vi "OSF Upload File.vi"(6 "Append to Lab Notebook":bool, 7 "timeout":dbl=60.0 format="%#_6ps", 8 "error in":errorcluster, 9 "Token":string, 10 "Node":string="96bhe/files/", 11 "File name":path=path "C:/Data/April_2019/042419/sp0006_042419.tdms") -> (0 "error out":errorcluster)   [LabVIEW 2020]
uses:
  <vilib>/httpClient/PUTFile.vi
  <vilib>/httpClient/PUTBuffer.vi
  <vilib>/httpClient/LabVIEWHTTPClient.lvlib
panel:
  in  "Export Type":enum16{"Text", "Markdown"}(ring)
  out "Elapsed time":dbl format="%#_6ps"
  out "body 2":string
  out "body":string
  in  "OSF API URL":string="https://api.osf.io/v2/"
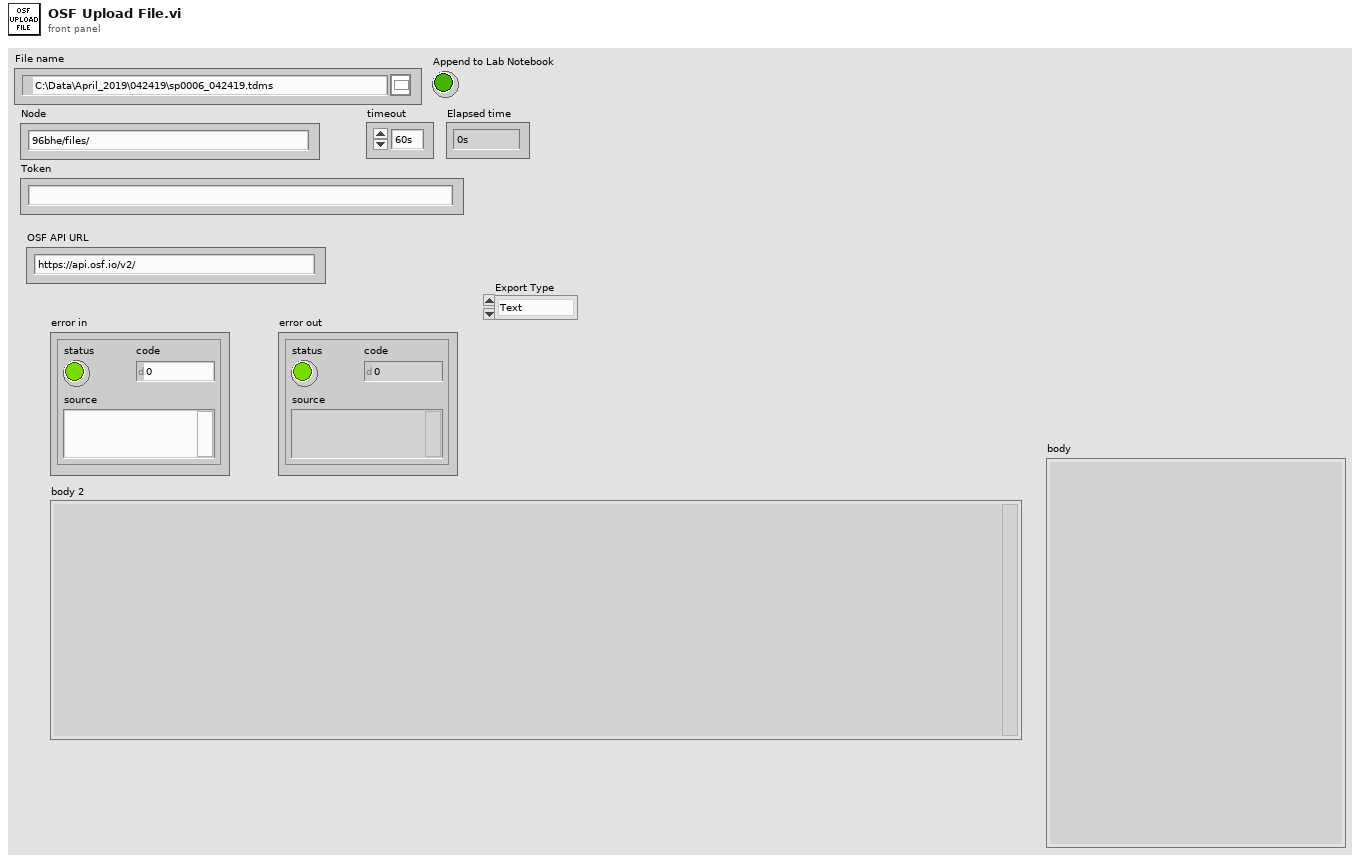
[diagram p1: front panel]
types:
  T1 = typedef "LabVIEWHTTPClient.lvlib/ClientHandle.ctl" = refnum<k1>
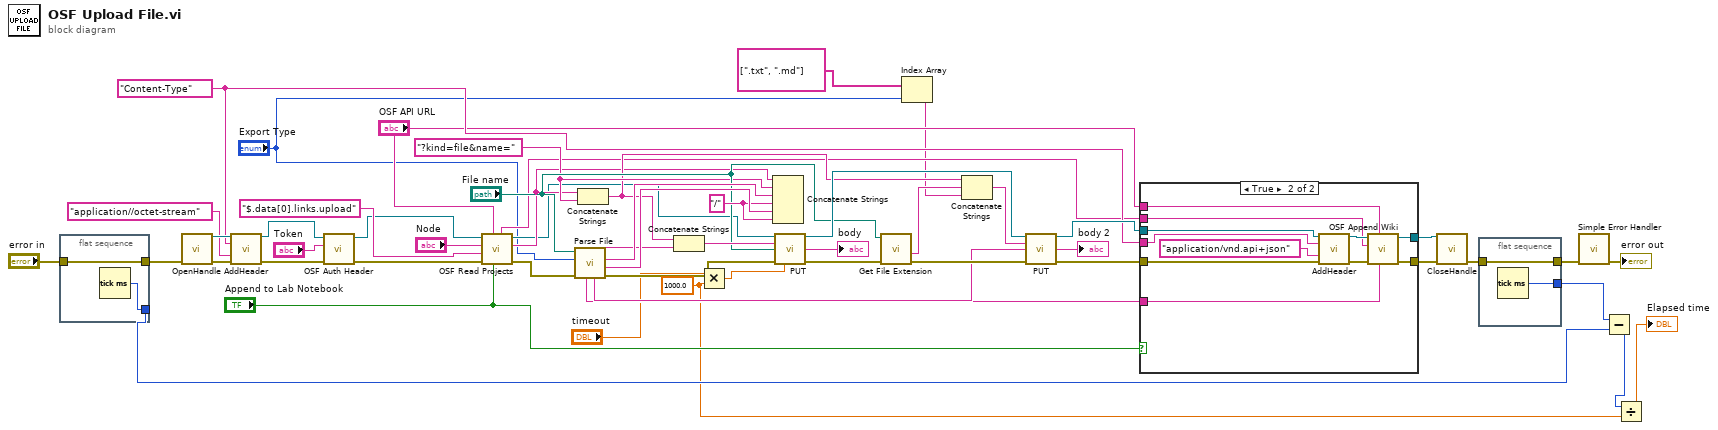
[diagram p0: block diagram]
diagram:
  w4 = 1000.0 ("y")
  w45 = "/" ("string")
  w33 = "?kind=file&name="
  w25 = "Content-Type" ("header")
  n1 = flat-sequence {
    tunnel: "error in" -> [w56]
    tunnel: [w56] -> w11
    tunnel: [w55] -> w7
    frame #0 {
      n2 = Tick Count (ms)() -> (millisecond timer value=w55:u32)
    }
  }
  n3 = call <vilib>:"OpenHandle.vi"("error in (no error)"=w11) -> ("client handle out"=w54:T1, "error out"=w53:errorcluster)  [unwired: 13 in]
  n4 = call <vilib>:"AddHeader.vi"("client handle"=w54, "header"=w25, "value"="application//octet-stream", "error in (no error)"=w53) -> ("client handle out"=w49:T1, "error out"=w20:errorcluster)  [unwired: 10 in]
  n5 = call "OSF Auth Header.vi"("error in"=w20, "Token"="Token", "client handle"=w49) -> ("error out"=w17:errorcluster, "client handle out"=w18:T1)  [unwired: 7 in]
  n6 = call "OSF Read Projects.vi"("Read wikis"="Append to Lab Notebook", "OSF API URL"="OSF API URL", "error in"=w17, "$Path or Item Name"="$.data[0].links.upload", "node"="Node", "client handle"=w18) -> ("error out"=w16:errorcluster, "Upload link"=w23:string, "client handle out"=w19:T1, "Wiki ID"=w22:string)  [unwired: 2 out]
  n7 = call "Parse File.vi"("error in"=w16, "Export Type"="Export Type", "File name"="File name") -> ("error out"=w44:errorcluster, "Dir 2"=w46:string, "Dir 1"=w47:string, "metadata"=w28:string, "File name"=w29:string, "Lab notebook entry"=w15:string)  [unwired: 1 in, 2 out]
  n8 = Concatenate Strings(w23, w33) -> (w32:string)
  n9 = Concatenate Strings(w32, w29) -> (w42:string)
  n10 = Multiply(x="timeout", y=w4) -> (x*y=w13:dbl)
  n11 = Concatenate Strings(w23, w33, w47, w45, w46, w45) -> ()  [unwired: 1 out]
  n12 = call-poly <vilib>:"PUT.vi"("client handle"=w19, "url"=w42, "file"="File name", "error in (no error)"=w44, "timeout (10000)"=w13) -> ("client handle out"=w43:T1, "body"=→"body":string, "error out"=w36:errorcluster)  [unwired: 7 in, 1 out]
  n13 = call <vilib>:"Get File Extension.vi"("error in (no error)"=w36, "file"="File name") -> ("error out"=w35:errorcluster, "filename without extension"=w40:string)  [unwired: 5 in, 3 out]
  n14 = Index Array(array=string[] [".txt", ".md"], index="Export Type") -> (element=w3:string)
  n15 = Concatenate Strings(w32, w40, w3) -> (w39:string)
  n16 = call-poly <vilib>:"PUT.vi"("client handle"=w43, "url"=w39, "buffer"=w28, "error in (no error)"=w35) -> ("client handle out"=w26:T1, "body"=→"body 2":string, "error out"=w27:errorcluster)  [unwired: 8 in, 1 out]
  n17 = case shown="True" "Append to Lab Notebook" {
    tunnel: [w57 w69] -> w31
    tunnel: [w58 w68] -> w30
    tunnel: w15 -> [_ w67]
    tunnel: w27 -> [w58 w66]
    tunnel: w26 -> [w57 w64]
    tunnel: w25 -> [_ w62]
    tunnel: "OSF API URL" -> [_ w60]
    tunnel: w22 -> [_ w59]
    frame False {
    }
    frame True {
      n18 = call <vilib>:"AddHeader.vi"("client handle"=w64, "header"=w62, "value"="application/vnd.api+json", "error in (no error)"=w66) -> ("client handle out"=w63:T1, "error out"=w65:errorcluster)  [unwired: 10 in]
      n19 = call "OSF Append Wiki.vi"("content"=w67, "OSF API URL"=w60, "error in"=w65, "Wiki  ID"=w59, "client handle"=w63) -> ("error out"=w68:errorcluster, "client handle out"=w69:T1)  [unwired: 4 in, 1 out]
    }
  }
  n20 = call <vilib>:"CloseHandle.vi"("client handle"=w31, "error in (no error)"=w30) -> ("error out"=w10:errorcluster)  [unwired: 13 in]
  n21 = flat-sequence {
    tunnel: w10 -> [w71]
    tunnel: [w71] -> w9
    tunnel: [w70] -> w8
    frame #0 {
      n22 = Tick Count (ms)() -> (millisecond timer value=w70:u32)
    }
  }
  n23 = call <vilib>:"Simple Error Handler.vi"("error in (no error)"=w9) -> ("error out"=→"error out":errorcluster)  [unwired: 4 in, 4 out]
  n24 = Subtract(x=w8, y=w7) -> (x-y=w5:u32)
  n25 = Divide(x=w5, y=w4) -> (x/y=→"Elapsed time":dbl)
